vi "Channel Basics Lesson 4.vi"() -> ()   [LabVIEW 2019]
doc: "This VI teaches users how to actually create a channel and how to replace one channel with another."
panel:
  in  "Stop Reader B":bool
  in  "Stop Writer B":bool
  out "Writer B":i32(graph)
  out "Reader B":i32(graph)
  # "Overview: This VI teaches users how to actually create a channel and how to replace one channel with another. \n\nInstructions:\n1. You will be editing this VI. Save a copy of it before you begin and edit the copy.\n2. Open the block diagram. Perform the editing instructions presented there."
  # "The terms \"Writer B\" and \"Reader B\" are retained because you will be learning how to replicate that section of Lesson 2. There is no \"A\" part in this lesson."
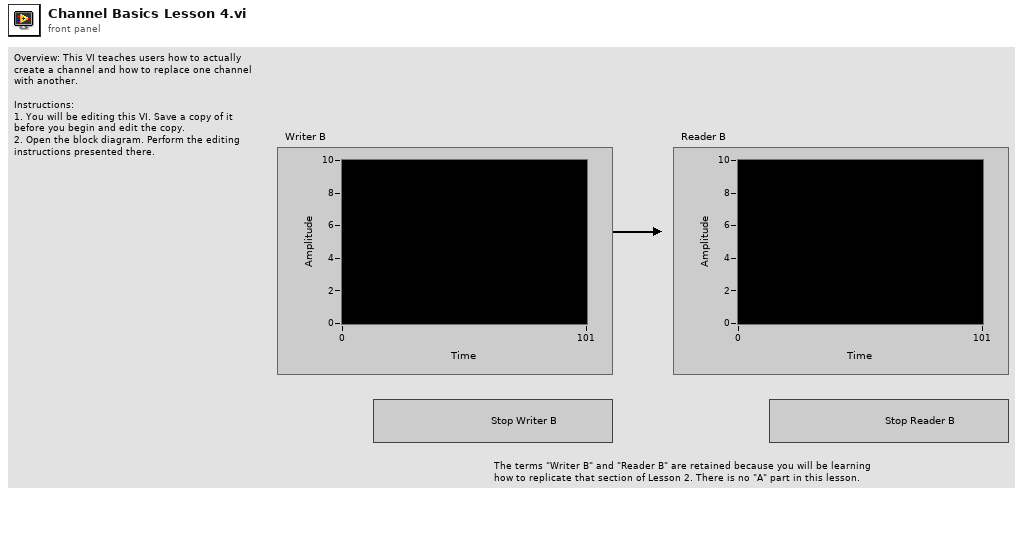
[diagram p1: front panel]
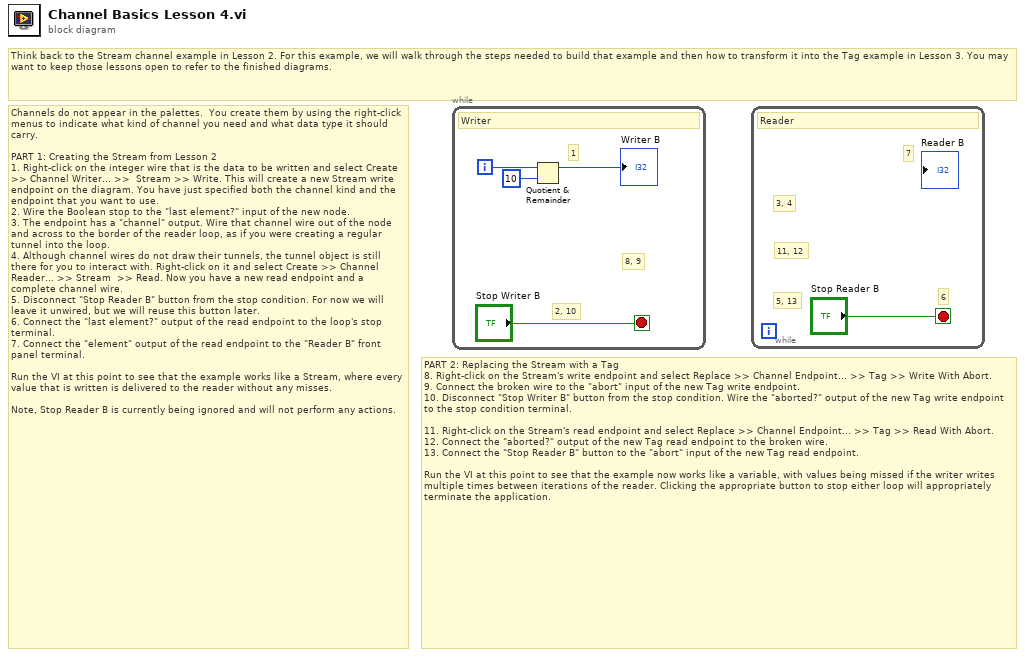
[diagram p0: block diagram]
diagram:
  # "PART 2: Replacing the Stream with a Tag\n8. Right-click on the Stream's write endpoint and select Replace >> Channel Endpoint... >> Tag >> Write With Abort.\n9. Connect the broken wire to the \"abort\" input of the new Tag write endpoint.\n10. Disconnect \"Stop Writer B\" button from the stop condition. Wire the \"aborted?\" output of the new Tag write endpoint to the stop condition terminal.\n\n11. Right-click on the Stream's read endpoint and select Replace >> Channel Endpoint... >> Tag >> Read With Abort.\n12. Connect the \"aborted?\" output of the new Tag read endpoint to the broken wire.\n13. Connect the \"Stop Reader B\" button to the \"abort\" input of the new Tag read endpoint.\n\nRun the VI at this point to see that the example now works like a variable, with values being missed if the writer writes multiple times between iterations of the reader. Clicking the appropriate button to stop either loop will appropriately terminate the application."
  # "Channels do not appear in the palettes.  You create them by using the right-click menus to indicate what kind of channel you need and what data type it should carry. \n\nPART 1: Creating the Stream from Lesson 2\n1. Right-click on the integer wire that is the data to be written and select Create >> Channel Writer... >>  Stream >> Write. This will create a new Stream write endpoint on the diagram. You have just specified both the channel kind and the endpoint that you want to use.\n2. Wire the Boolean stop to the \"last element?\" input of the new node.\n3. The endpoint has a \"channel\" output. Wire that channel wire out of the node and across to the border of the reader loop, as if you were creating a regular tunnel into the loop. \n4. Although channel wires do not draw their tunnels, the tunnel object is still there for you to interact with. Right-click on it and select Create >> Channel Reader... >> Stream  >> Read. Now you have a new read endpoint and a complete channel wire.\n5. Disconnect \"Stop Reader B\" button from the stop condition. For now we will leave it unwired, but we will reuse this button later.\n6. Connect the \"last element?\" output of the read endpoint to the loop's stop terminal. \n7. Connect the \"element\" output of the read endpoint to the \"Reader B\" front panel terminal.\n\nRun the VI at this point to see that the example works like a Stream, where every value that is written is delivered to the reader without any misses.\n\nNote, Stop Reader B is currently being ignored and will not perform any actions."
  # "Think back to the Stream channel example in Lesson 2. For this example, we will walk through the steps needed to build that example and then how to transform it into the Tag example in Lesson 3. You may want to keep those lessons open to refer to the finished diagrams."
  n1 = while {
    i -> [w3]
    stop <- "Stop Writer B" stop-if-true
    # "8, 9"
    # "2, 10"
    # "1"
    # "Writer"
    n2 = Quotient & Remainder(x=w3, y=10) -> (x-y*floor(x/y)=→"Writer B":i32)  [unwired: 1 out]
  }
  n3 = while {
    stop <- "Stop Reader B" stop-if-true
    # "11, 12"
    # "7"
    # "6"
    # "5, 13"
    # "3, 4"
    # "Reader"
  }
